vi "select_form_field.vi"(10 "Name":string, 11 "Form Data":T1[](array[typedef])) -> (2 "not found":bool, 3 "Form Data":T1[](array[typedef]))   [LabVIEW 2011]
uses:
  html_form_field.ctl
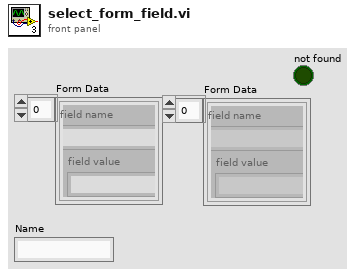
[diagram p1: front panel]
types:
  T1 = typedef "html_form_field.ctl" = cluster{"field name":string, "field value":string}
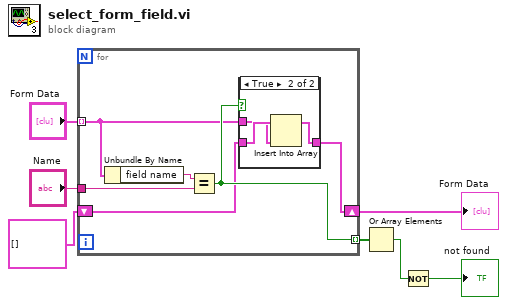
[diagram p0: block diagram]
diagram:
  n1 = for {
    tunnel: "Form Data" -> [w10] mode=indexing
    tunnel: "Name" -> [w12]
    tunnel: [w11] -> w5 mode=indexing
    shift-right: [w8] -> w1
    shift-left: T1[] [] -> [w9]
    n2 = Unbundle By Name(w10) -> ("field name"=w13:string)
    n3 = Equal?(x=w13, y=w12) -> (x = y?=w11:bool)
    n4 = case shown="True" w11 {
      tunnel: w10 -> [_ w16]
      tunnel: w9 -> [w14 w17]
      tunnel: [w14 w15] -> w8
      frame False {
      }
      frame True {
        n5 = Insert Into Array(array=w17, new element=w16) -> (w15:T1[])  [unwired: 1 in]
      }
    }
  }
  "Form Data" <- w1
  n6 = Or Array Elements(Boolean array=w5) -> (logical OR=w3:bool)
  n7 = Not(x=w3) -> (.not. x?=→"not found":bool)
